vi "Open_1D_Selection.vi"(0 "path":path=path "C:/misc/LabVIEW/FILES/1D_array(col).psv", 2 "delimiter":string="|", 4 "index":i32, 5 "Row/Col":enum16{"Row", "Col"}(ring)=enum."Col") -> (16 "1D Sub Array":dbl[](array[numeric])=[0.00033432, 0.0, 0.0, 3.432e-05] format="%.6f")   [LabVIEW 2014]
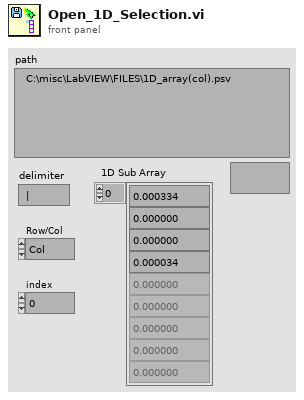
[diagram p1: front panel]
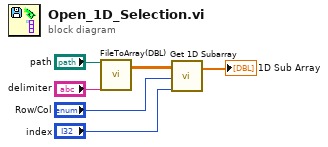
[diagram p0: block diagram]
diagram:
  n1 = call "FileToArray(DBL).vi"("path"="path", "delimiter"="delimiter") -> ("data"=w6:dbl[][])  [unwired: 15 in, 2 out]
  n2 = call "Get 1D Subarray.vi"("2D Array"=w6, "Row/Col"="Row/Col", "index"="index") -> ("1D Sub Array"=→"1D Sub Array":dbl[])  [unwired: 16 in]
